vi "LVObject to JSON - True - Pretty Print Enabled.vi"() -> ()   [LabVIEW 2017, in "Generic Object Serializer Tests.lvlib" / "Pretty Print.lvlib"]
uses:
  Pretty Print.lvlib
  Generic Object Serializer/Generic Object Serializer.lvclass
  <vilib>/addons/_JKI Toolkits/Caraya/classes/Assert/Assert Equal Value_Variant.vi
  <vilib>/addons/_JKI Toolkits/Caraya/classes/Test/Test.lvclass
  <vilib>/addons/_JKI Toolkits/Caraya/classes/Assert/Assert.lvclass
  Temperature Forecast/Temperature Forecast.lvclass
panel:
  out "error out":errorcluster
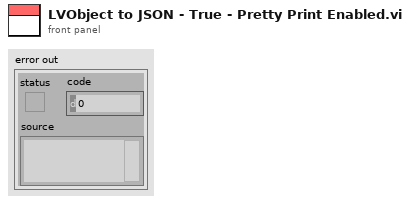
[diagram p1: front panel]
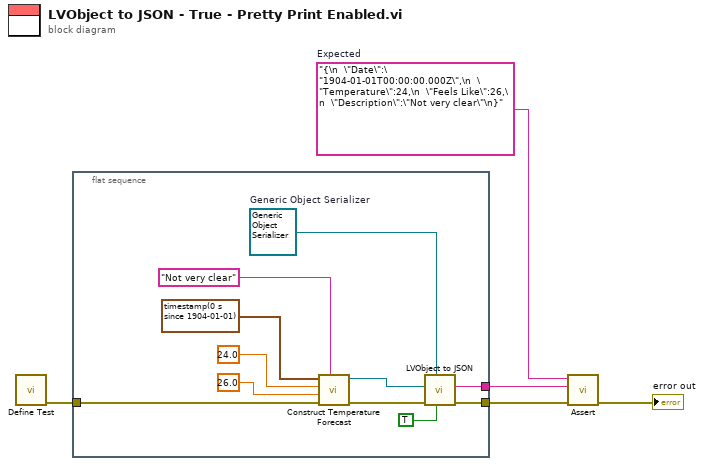
[diagram p0: block diagram]
diagram:
  w1 = "{\n  \"Date\":\"1904-01-01T00:00:00.000Z\",\n  \"Temperature\":24,\n  \"Feels Like\":26,\n  \"Description\":\"Not very clear\"\n}"  # Expected
  n1 = call <vilib>:"Define Test.vi"() -> ("error out"=w4:errorcluster)  [unwired: 11 in]
  n2 = flat-sequence {
    tunnel: w4 -> [w9]
    tunnel: [w15] -> w3
    tunnel: [w14] -> w2
    frame #0 {
      w16 = refnum<class "Generic Object Serializer.lvclass"> refnum  # Generic Object Serializer
      n3 = call "Construct Temperature Forecast.vi"("Description"="Not very clear", "error in (no error)"=w9, "Feels Like [°C]"=26.0, "Temperature [°C]"=24.0, "Date"=timestamp(0 s since 1904-01-01)) -> ("error out"=w8:errorcluster, "Temperature Forecast"=w7:refnum<class "Temperature Forecast.lvclass">)  [unwired: 5 in]
      n4 = call-dynamic "LVObject to JSON.vi"("Pretty Print?"=TRUE, "LVClass Serializer"=w16, "error in (no error)"=w8, "Object"=w7) -> ("error out"=w15:errorcluster, "<JSON>Object"=w14:string)  [unwired: 6 in]
    }
  }
  n5 = call-poly <vilib>:"Assert.vi"("error in (no error)"=w3, "Y"=w2, "X"=w1) -> ("error out"=→"error out":errorcluster)  [unwired: 8 in]
